vi "NetworkCommand.Handler.vi"(8 "error in (no error)":errorcluster, 11 "J1939 Main Configuration":T1) -> (0 "error out":errorcluster)   [LabVIEW 2015, in "J1939 Addon Engine.lvlib"]
uses:
  J1939 Addon Engine.lvlib
  Types/Protocol.Configuration.ctl
  <vilib>/NI/NIVS Addon Network Comm/Engine/VeriStand Comm.lvclass
  <vilib>/NI/NIVS Inline Async API/_VS Inline Async API/Process/Process.lvclass
  Types/Protocol.Refs.ctl
  Shared/J1939 Utilities/Types/CAN Outgoing Message Cluster.ctl
  Types/Protocol.RQST Lookup Table Reference.ctl
  Types/Protocol.Address Table Reference.ctl
  Types/Protocol.XNET Settings.ctl
  <vilib>/NI/NIVS Addon Network Comm/Engine/VeriStand Comm.lvclass/VeriStand Comm.ctl
  Shared/Types/Request Message.ctl
  Types/Protocol.Address Lookup Table Action.ctl
  <vilib>/NI/NIVS Inline Async API/_VS Inline Async API/Process/Process.lvclass/Process.ctl
  <vilib>/NI/NIVS Inline Async API/_VS Inline Async API/Error Handling Process/SubVIs/Error.ConvertArray.vi
  <vilib>/NI/AMC/Read Next Message.vi
  <vilib>/NI/Tools/Keyed Array/Index.vi
  Shared/J1939 Utilities/Common Messages.vi
  Shared/J1939 Utilities/SubVIs/Request.vi
  Protocol.RQST Lookup Table Act.vi
  <vilib>/NI/AMC/Send Local Message.vi
  <vilib>/NI/AMC/Read Termination Message.vi
  <vilib>/NI/Tools/Keyed Array/Map String.vi
  Shared/J1939 Utilities/Common Conversions.vi
  Shared/J1939 Utilities/SubVIs/Convert J1939 ID to CAN Arb ID.vi
  <vilib>/NI/AMC/Create Single Message.vi
  <vilib>/NI/AMC/Update Message Routing Info.vi
  <vilib>/NI/Tools/String/Get Case Matching.vi
  <vilib>/NI/AMC/Send Message.vi
  Protocol.Address Lookup Table.vi
  <vilib>/xnet/xnet.llb/XNET Read (State CAN Comm).vi
  Protocol.RQST Lookup Table.vi
  <vilib>/NI/AMC/Globals.vi
  <vilib>/NI/NIVS Addon Network Comm/Shared/Comm Constants.vi
  Shared/J1939 Addon Shared.lvlib
  Shared/J1939 Utilities/J1939 Utilities.lvlib
  <vilib>/NI Veristand/Custom Device Tools/Custom Device Utility Library/Custom Device Utility Library.lvlib
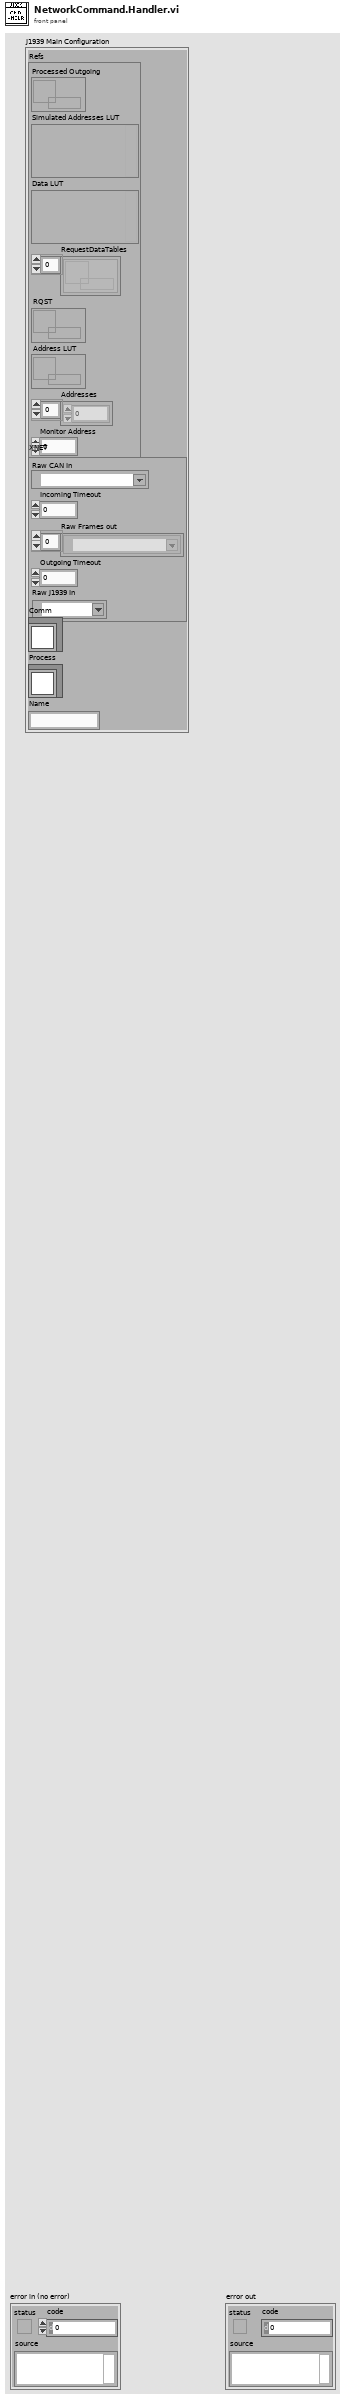
[diagram p1: front panel]
types:
  T1 = typedef "J1939 Addon Engine.lvlib/Protocol.Configuration.ctl" = cluster{"Refs":T2, "XNET":T5, "Comm":refnum<class "VeriStand Comm.lvclass">, "Process":refnum<class "Process.lvclass">, "Name":string}
  T2 = typedef "J1939 Addon Engine.lvlib/Protocol.Refs.ctl" = cluster{"Processed Outgoing":refnum<queue>, "Simulated Addresses LUT":variant, "Data LUT":variant, "RequestDataTables":refnum<k33>[], "RQST":T3, "Address LUT":T4, "Addresses":u8[], "Monitor Address":u8}
  T3 = typedef "J1939 Addon Engine.lvlib/Protocol.RQST Lookup Table Reference.ctl" = refnum<data-value>
  T4 = typedef "J1939 Addon Engine.lvlib/Protocol.Address Table Reference.ctl" = refnum<data-value>
  T5 = typedef "J1939 Addon Engine.lvlib/Protocol.XNET Settings.ctl" = cluster{"Raw CAN In":refnum<k21>, "Incoming Timeout":u32, "Raw Frames out":refnum<k21>[], "Outgoing Timeout":u32, "Raw J1939 In":refnum<k21>}
  T6 = typedef "J1939 Addon Shared.lvlib/Request Message.ctl" = cluster{"PGN":u32, "DA":u8, "Ignore Response":bool}
  T7 = typedef "J1939 Addon Shared.lvlib/J1939 Utilities.lvlib/CAN Outgoing Message Cluster.ctl" = cluster{"Identifier":u32, "Data":u8[]}
  T8 = typedef "J1939 Addon Engine.lvlib/Protocol.Address Lookup Table Action.ctl" = enum16{"Initialize", "Add", "Get", "Remove", "Get All"}
  T9 = typedef "NI VeriStand Addon Network Comm.lvlib/VeriStand Comm.lvclass/Response Information.ctl" = cluster{"response name":string, "responseQ":string}
  T10 = typedef "XNET Frame CAN.ctl" = cluster{"timestamp":timestamp, "payload":u8[], "identifier":u32, "type":T11, "extended?":bool, "echo?":bool}
  T11 = typedef "XNET Frame Type CAN.ctl" = u8
  T12 = typedef "XNET CAN Comm.ctl" = cluster{"fault code":i32, "fault?":bool, "communication state":T13, "last error":T14, "receive error counter":u8, "transmit error counter":u8, "transceiver error?":bool, "sleep?":bool}
  T13 = typedef "XNET CAN Comm State.ctl" = u8
  T14 = typedef "XNET CAN Last Err.ctl" = u8
  T15 = typedef "J1939 Addon Shared.lvlib/Address Lookup Table Data.ctl" = cluster{"Name":u8[], "Address":u8}
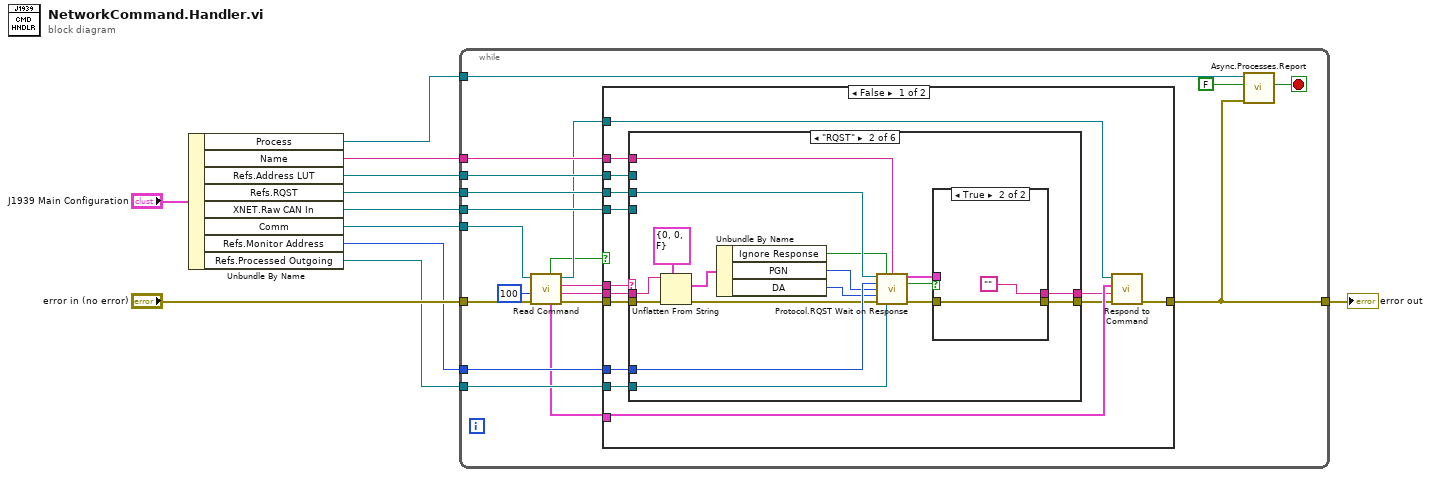
[diagram p0: block diagram]
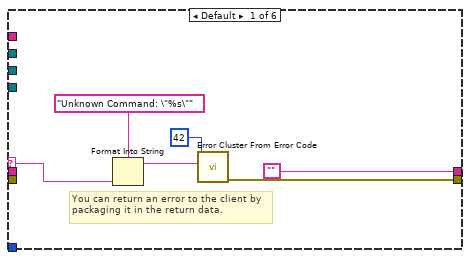
[diagram p2: hidden frame]
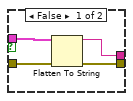
[diagram p3: hidden frame]
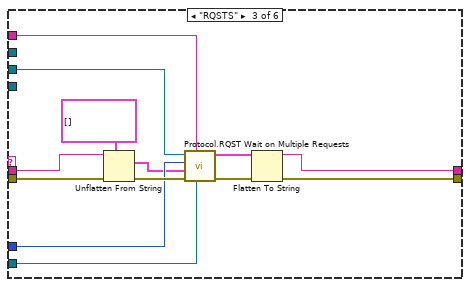
[diagram p4: hidden frame]
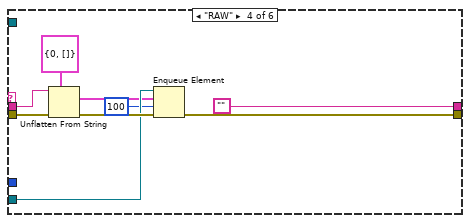
[diagram p5: hidden frame]
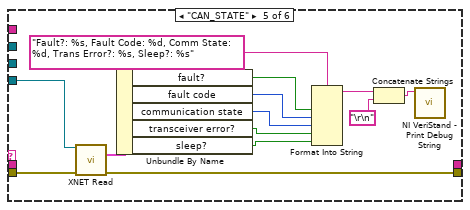
[diagram p6: hidden frame]
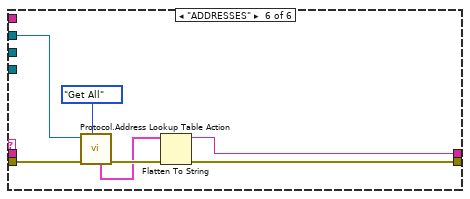
[diagram p7: hidden frame]
diagram:
  n1 = Unbundle By Name("J1939 Main Configuration") -> ("Process"=w2:refnum<class "Process.lvclass">, "Name"=w3:string, "Refs.Address LUT"=w4:T4, "Refs.RQST"=w5:T3, "XNET.Raw CAN In"=w6:refnum<k21>, "Comm"=w7:refnum<class "VeriStand Comm.lvclass">, "Refs.Monitor Address"=w8:u8, "Refs.Processed Outgoing"=w9:refnum<queue>)
  n2 = while {
    tunnel: "error in (no error)" -> [w27]
    tunnel: [w19] -> w10
    tunnel: w2 -> [w29]
    tunnel: w7 -> [w26]
    tunnel: w3 -> [w25]
    tunnel: w6 -> [w24]
    tunnel: w9 -> [w23]
    tunnel: w8 -> [w22]
    tunnel: w5 -> [w21]
    tunnel: w4 -> [w20]
    stop <- w30 stop-if-true
    n3 = call <vilib>:"Read Command.vi"("error in (no error)"=w27, "timeout (100 ms)"=100, "VeriStand Comm in"=w26) -> ("error out"=w17:errorcluster, "message value"=w15:string, "message name"=w16:string, "VeriStand Comm out"=w13:refnum<class "VeriStand Comm.lvclass">, "ResponseInfo"=w14:T9, "timed out?"=w12:bool)  [unwired: 3 in]
    n4 = case shown="False" w12 {
      tunnel: w25 -> [w44 _]
      tunnel: w24 -> [w43 _]
      tunnel: w23 -> [w42 _]
      tunnel: w22 -> [w41 _]
      tunnel: w21 -> [w40 _]
      tunnel: w20 -> [w39 _]
      tunnel: [w38 w116] -> w19
      tunnel: w17 -> [w37 w116]
      tunnel: w16 -> [w36 _]
      tunnel: w15 -> [w35 _]
      tunnel: w14 -> [w34 _]
      tunnel: w13 -> [w33 _]
      frame False {
        n5 = case shown="\"RQST\"" w36 {
          selector: w36 -> [w46 _ _ _ _ _]
          tunnel: w35 -> [_ w54 w83 w94 _ _]
          tunnel: [w47 w66 w86 w88 w106 w109] -> w31
          tunnel: ["" ("data string") w63 w85 "" _ w110] -> w32
          tunnel: w42 -> [_ w61 w80 w91 _ _]
          tunnel: w37 -> [_ w60 w84 w95 w108 w114]
          tunnel: w40 -> [_ w53 w78 _ _ _]
          tunnel: w41 -> [_ w67 w77 _ _ _]
          tunnel: w39 -> [_ _ _ _ _ w113]
          tunnel: w44 -> [_ w51 w74 _ _ _]
          tunnel: w43 -> [_ _ _ _ w107 _]
          frame Default {
            # "You can return an error to the client by packaging it in the return data."
            n6 = Format Into String(format string="Unknown Command: \"%s\"", w46) -> (resulting string=w48:string)  [unwired: 2 in, 1 out]
            n7 = call <vilib>:"Error Cluster From Error Code.vi"("error message (\"\")"=w48, "error code (0)"=42) -> ("error out"=w47:errorcluster)  [unwired: 7 in]
          }
          frame "RQST" {
            n8 = Unflatten From String(type=T6 {"PGN"=0, "DA"=0, "Ignore Response"=FALSE} ("Cluster"), binary string=w54, error in (no error)=w60) -> (value=w57:T6, error out=w59:errorcluster)  [unwired: 2 in, 1 out]
            n9 = Unbundle By Name(w57) -> ("Ignore Response"=w52:bool, "PGN"=w56:u32, "DA"=w55:u8)
            n10 = call "Protocol.RQST Wait on Response.vi"("ref in"=w53, "Ignore Response"=w52, "Name"=w51, "Source Address"=w67, "PGN"=w56, "DA"=w55, "error in (no error)"=w59, "Processed Outgoing"=w61) -> ("element"=w62:T10, "timed out?"=w64:bool, "error out"=w65:errorcluster)  [unwired: 4 in, 1 out]
            n11 = case shown="True" w64 {
              tunnel: [w69 w73] -> w66
              tunnel: w65 -> [w70 w73]
              tunnel: [w68 ""] -> w63
              tunnel: w62 -> [w71 _]
              frame False {
                n12 = Flatten To String(anything=w71, error in (no error)=w70) -> (data string=w68:string, error out=w69:errorcluster)  [unwired: 2 in, 1 out]
              }
              frame True {
              }
            }
          }
          frame "RQSTS" {
            n13 = Unflatten From String(type=T6[] [], binary string=w83, error in (no error)=w84) -> (value=w76:T6[], error out=w81:errorcluster)  [unwired: 2 in, 1 out]
            n14 = call "Protocol.RQST Wait on Multiple Requests.vi"("Processed Outgoing"=w80, "Name"=w74, "error in (no error)"=w81, "value"=w76, "Source Address"=w77, "ref in"=w78) -> ("error out"=w79:errorcluster, "Elements"=w75:T10[])  [unwired: 2 in, 2 out]
            n15 = Flatten To String(anything=w75, error in (no error)=w79) -> (data string=w85:string, error out=w86:errorcluster)  [unwired: 2 in, 1 out]
          }
          frame "RAW" {
            n16 = Unflatten From String(type=T7 {"Identifier"=0, "Data"=[]} ("Data to Send"), binary string=w94, error in (no error)=w95) -> (value=w90:T7, error out=w92:errorcluster)  [unwired: 2 in, 1 out]
            n17 = Enqueue Element(queue=w91, element=w90, timeout in ms (-1)=100, error in (no error)=w92) -> (error out=w88:errorcluster)  [unwired: 2 out]
          }
          frame "CAN_STATE" {
            n18 = call-poly <vilib>:"XNET Read.vi"("session in"=w107, "error in (no error)"=w108) -> ("CAN comm"=w105:T12, "error out"=w106:errorcluster)  [unwired: 11 in, 1 out]
            n19 = Unbundle By Name(w105) -> ("fault?"=w104:bool, "fault code"=w103:i32, "communication state"=w102:T13, "transceiver error?"=w101:bool, "sleep?"=w100:bool)
            n20 = Format Into String(format string="Fault?: %s, Fault Code: %d, Comm State: %d, Trans Error?: %s, Sleep?: %s", w104, w103, w102, w101, w100) -> (resulting string=w99:string)  [unwired: 2 in, 1 out]
            n21 = Concatenate Strings(w99, "\r\n") -> (w97:string)
            n22 = call <vilib>:"NI VeriStand - Print Debug String.vi"("Message"=w97) -> ()  [unwired: 10 in, 1 out]
          }
          frame "ADDRESSES" {
            n23 = call "Protocol.Address Lookup Table Action.vi"("Action"=Protocol.Address_Lookup_Table_Action."Get All", "error in (no error)"=w114, "ref in"=w113) -> ("error out"=w112:errorcluster, "All Data"=w111:T15[])  [unwired: 5 in, 2 out]
            n24 = Flatten To String(anything=w111, error in (no error)=w112) -> (data string=w110:string, error out=w109:errorcluster)  [unwired: 2 in, 1 out]
          }
        }
        n25 = call <vilib>:"Respond to Command.vi"("error in (no error)"=w31, "message value"=w32, "ResponseInfo"=w34, "VeriStand Comm in"=w33) -> ("error out"=w38:errorcluster)  [unwired: 5 in, 2 out]
      }
      frame True {
      }
    }
    n26 = call <vilib>:"Async.Processes.Report.vi"("Error"=w19, "Stop Async on Error?"=FALSE ("Stop on Error?"), "Process in"=w29) -> ("Stop"=w30:bool)  [unwired: 7 in, 1 out]
  }
  "error out" <- w10
